vi "Read and Check Faults - Debug.vi"(8 "error in (no error)":errorcluster, 9 "JSONCluster":T1 {"DMMVoltageFaultUpperLimit" format="%#_6p"}, 10 "DMM Ref":refnum<k15>, 11 "SMU Ref":refnum<k15>) -> (0 "error out":errorcluster, 1 "Result":T2, 2 "DMM Ref Out":refnum<k15>, 3 "SMU Ref Out":refnum<k15>)   [LabVIEW 2019]
uses:
  labview-grpc-query-server/VIs/MeasurementServer_FourProbeRawData.ctl
  labview-grpc-query-server/VIs/MeasurementServer_ErrorOutData.ctl
  JSONCluster.ctl
  labview-grpc-query-server/VIs/labview-grpc-measurement-server.lvlib
  SupportVIs.lvlib
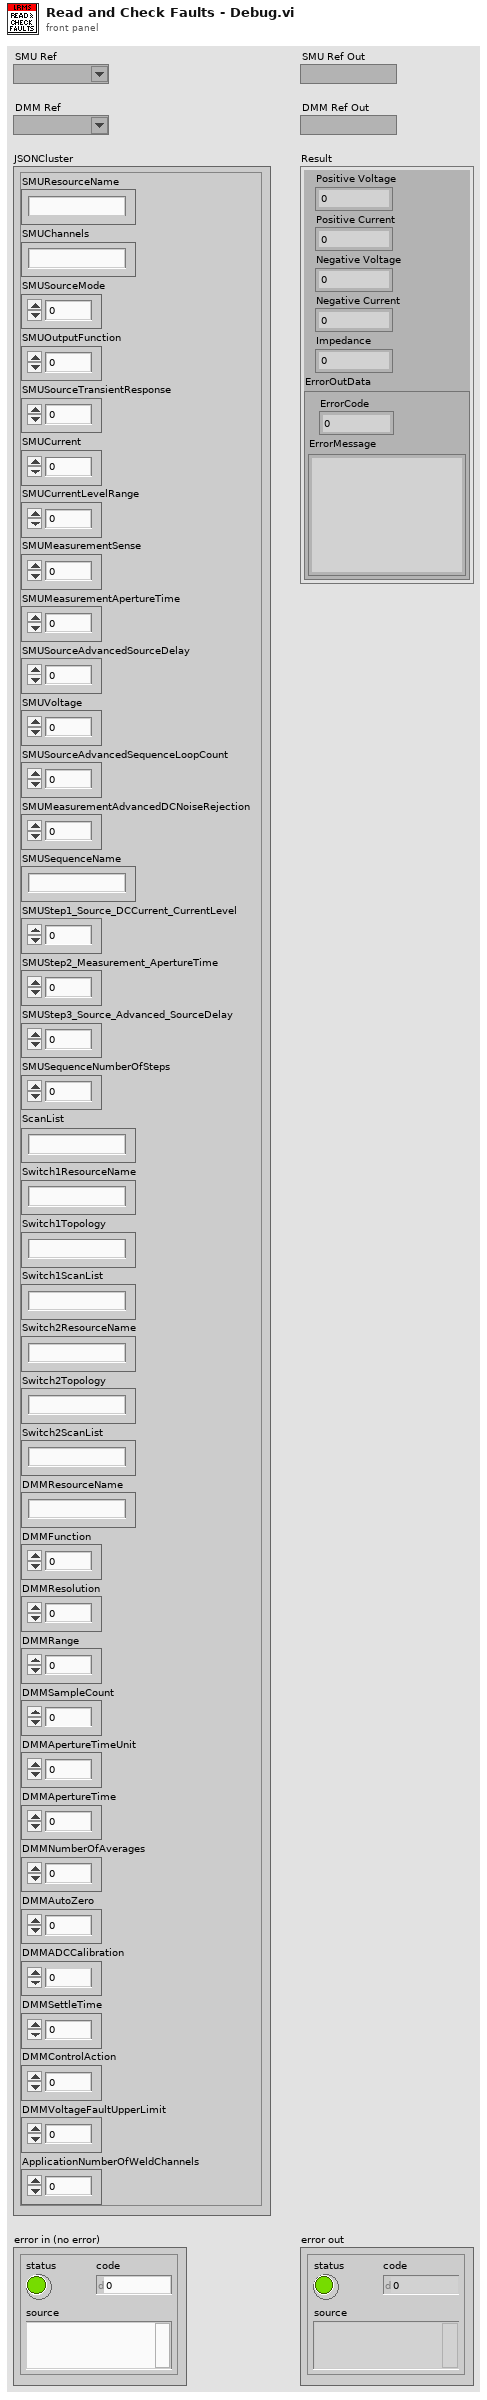
[diagram p1: front panel]
types:
  T1 = typedef "JSONCluster.ctl" = cluster{"SMUResourceName":string, "SMUChannels":string, "SMUSourceMode":i32, "SMUOutputFunction":i32, "SMUSourceTransientResponse":i32, "SMUCurrent":dbl, "SMUCurrentLevelRange":dbl, "SMUMeasurementSense":i32, "SMUMeasurementApertureTime":dbl, "SMUSourceAdvancedSourceDelay":dbl, "SMUVoltage":dbl, "SMUSourceAdvancedSequenceLoopCount":i32, "SMUMeasurementAdvancedDCNoiseRejection":i32, "SMUSequenceName":string, "SMUStep1_Source_DCCurrent_CurrentLevel":i32, "SMUStep2_Measurement_ApertureTime":i32, "SMUStep3_Source_Advanced_SourceDelay":i32, "SMUSequenceNumberOfSteps":i32, "ScanList":string, "Switch1ResourceName":string, "Switch1Topology":string, "Switch1ScanList":string, "Switch2ResourceName":string, "Switch2Topology":string, "Switch2ScanList":string, "DMMResourceName":string, "DMMFunction":i32, "DMMResolution":dbl, "DMMRange":dbl, "DMMSampleCount":i32, "DMMApertureTimeUnit":i32, "DMMApertureTime":dbl, "DMMNumberOfAverages":i32, "DMMAutoZero":i32, "DMMADCCalibration":i32, "DMMSettleTime":dbl, "DMMControlAction":i32, "DMMVoltageFaultUpperLimit":dbl, "ApplicationNumberOfWeldChannels":i32}
  T2 = typedef "labview-grpc-measurement-server.lvlib/MeasurementServer_FourProbeRawData.ctl" = cluster{"Positive Voltage":dbl, "Positive Current":dbl, "Negative Voltage":dbl, "Negative Current":dbl, "Impedance":dbl, "ErrorOutData":T3}
  T3 = typedef "labview-grpc-measurement-server.lvlib/MeasurementServer_ErrorOutData.ctl" = cluster{"ErrorCode":i32, "ErrorMessage":string}
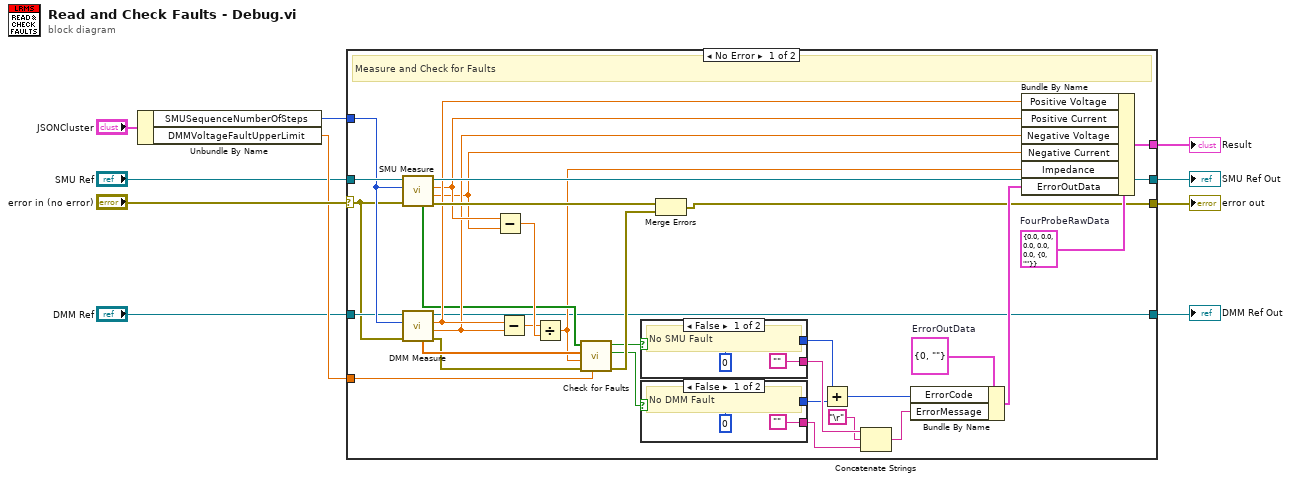
[diagram p0: block diagram]
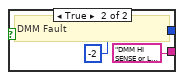
[diagram p2: hidden frame]
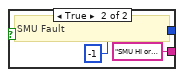
[diagram p3: hidden frame]
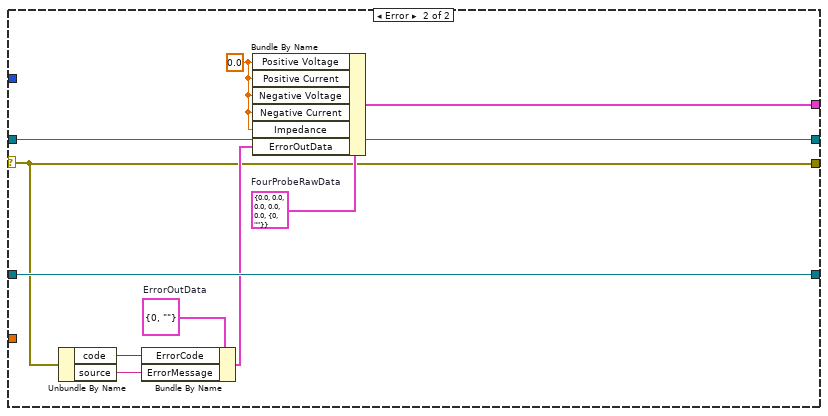
[diagram p4: hidden frame]
diagram:
  n1 = Unbundle By Name("JSONCluster") -> ("SMUSequenceNumberOfSteps"=w3:i32, "DMMVoltageFaultUpperLimit"=w7:dbl)
  n2 = case shown="No Error" "error in (no error)" {
    selector: "error in (no error)" -> [w12 w53]
    tunnel: [w43 w61] -> w1
    tunnel: [w19 w54] -> w10
    tunnel: "SMU Ref" -> [w18 w61]
    tunnel: w3 -> [w17 _]
    tunnel: "DMM Ref" -> [w16 w60]
    tunnel: [w14 w60] -> w2
    tunnel: w7 -> [w13 _]
    tunnel: [w11 w53] -> w4
    frame No Error {
      w21 = T3 {"ErrorCode"=0, "ErrorMessage"=""}  # ErrorOutData
      w20 = T2 {"Positive Voltage"=0.0, "Positive Current"=0.0, "Negative Voltage"=0.0, "Negative Current"=0.0, "Impedance"=0.0, "ErrorOutData"={"ErrorCode"=0, "ErrorMessage"=""}}  # FourProbeRawData
      # "Measure and Check for Faults"
      n3 = call "SMU Measure.vi"("error in (no error)"=w12, "SMUSequenceNumberOfSteps"=w17, "IVI Refnum in"=w18) -> ("error out"=w42:errorcluster, "Numeric"=w35:dbl, "Numeric 2"=w37:dbl, "IVI Refnum out"=w43:refnum<k15>, "in compliance"=w24:bool[])  [unwired: 4 in]
      n4 = call "DMM Measure.vi"("error in (no error)"=w12, "SMUSequenceNumberOfSteps"=w17, "IVI Refnum in"=w16) -> ("error out"=w15:errorcluster, "Numeric"=w36:dbl, "Numeric 2"=w38:dbl, "IVI Refnum out"=w14:refnum<k15>, "Measurements"=w23:dbl[])  [unwired: 4 in]
      n5 = Subtract(x=w37, y=w35) -> (x-y=w40:dbl)
      n6 = Subtract(x=w38, y=w36) -> (x-y=w39:dbl)
      n7 = Divide(x=w39, y=w40) -> (x/y=w22:dbl)
      n8 = call "Check for Faults.vi"("DMM Voltage Fault Upper Limit"=w13, "Error In"=w15, "Resistance In"=w22, "dmm voltage measurements"=w23, "in compliance"=w24) -> ("Error Out"=w41:errorcluster, "DMM Fault"=w28:bool, "SMU Fault"=w32:bool)  [unwired: 3 in, 1 out]
      n9 = case shown="False" w32 {
        tunnel: ["" "SMU HI or LO lead disconnected\n- SMU in compliance\n- SMU Fault = True"] -> w31
        tunnel: [0 -1] -> w29
        frame False {
          # "No SMU Fault"
        }
        frame True {
          # "SMU Fault"
        }
      }
      n10 = case shown="False" w28 {
        tunnel: ["" "DMM HI SENSE or LO SENSE lead disconnected\n- DMM measures NaN, or \n- DMM overrange warning, or\n- DMM voltage > 50uV "] -> w26
        tunnel: [0 -2] -> w25
        frame False {
          # "No DMM Fault"
        }
        frame True {
          # "DMM Fault"
        }
      }
      n11 = Merge Errors(w42, w41) -> (w11:errorcluster)
      n12 = Add(x=w29, y=w25) -> (x+y=w33:i32)
      n13 = Concatenate Strings(w31, "\r", w26) -> (w30:string)
      n14 = Bundle By Name(cluster=w21, "ErrorCode"=w33, "ErrorMessage"=w30) -> (w34:T3)
      n15 = Bundle By Name(cluster=w20, "Positive Voltage"=w38, "Positive Current"=w37, "Negative Voltage"=w36, "Negative Current"=w35, "Impedance"=w22, "ErrorOutData"=w34) -> (w19:T2)
    }
    frame Error {
      w52 = 0.0 ("Positive Voltage")
      w57 = T3 {"ErrorCode"=0, "ErrorMessage"=""}  # ErrorOutData
      w58 = T2 {"Positive Voltage"=0.0, "Positive Current"=0.0, "Negative Voltage"=0.0, "Negative Current"=0.0, "Impedance"=0.0, "ErrorOutData"={"ErrorCode"=0, "ErrorMessage"=""}}  # FourProbeRawData
      n16 = Unbundle By Name(w53) -> ("code"=w55:i32, "source"=w56:string)
      n17 = Bundle By Name(cluster=w57, "ErrorCode"=w55, "ErrorMessage"=w56) -> (w59:T3)
      n18 = Bundle By Name(cluster=w58, "Positive Voltage"=w52, "Positive Current"=w52, "Negative Voltage"=w52, "Negative Current"=w52, "Impedance"=w52, "ErrorOutData"=w59) -> (w54:T2)
    }
  }
  "Result" <- w10
  "error out" <- w4
  "DMM Ref Out" <- w2
  "SMU Ref Out" <- w1
